vi "Delete FITS.vi"(8 "error in (no error)":errorcluster, 11 "Save Image in":refnum<class "Save Image.lvclass">) -> (0 "error out":errorcluster, 3 "Save Image out":refnum<class "Save Image.lvclass">)   [LabVIEW 2018, in "Save Image.lvclass"]
uses:
  Save Image.lvclass
  Save Image.lvclass/Save Image.ctl
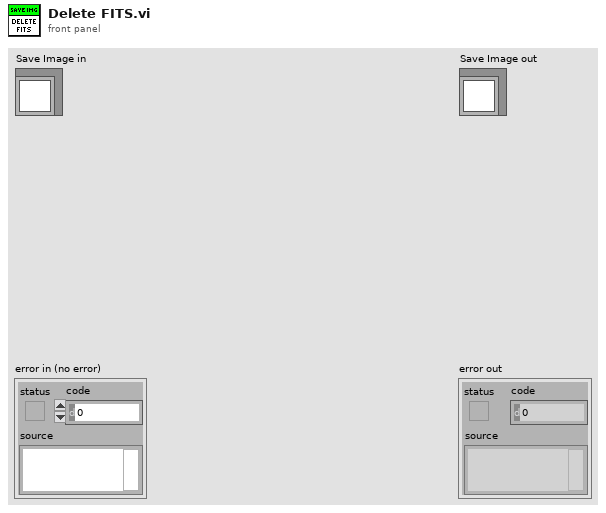
[diagram p1: front panel]
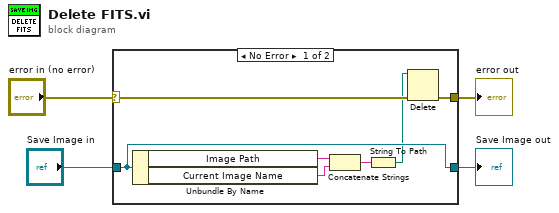
[diagram p0: block diagram]
diagram:
  n1 = case shown="No Error" "error in (no error)" {
    selector: "error in (no error)" -> [w10 w13]
    tunnel: [w9 w13] -> w3
    tunnel: [w11 w12] -> w1
    tunnel: "Save Image in" -> [w11 w12]
    frame No Error {
      n2 = Unbundle By Name(w11) -> ("Image Path"=w7:string, "Current Image Name"=w8:string)
      n3 = Concatenate Strings(w7, w8) -> (w6:string)
      n4 = String To Path(string=w6) -> (path=w5:path)
      n5 = Delete(path (use dialog)=w5, error in=w10) -> (error out=w9:errorcluster)  [unwired: 3 in, 2 out]
    }
    frame Error {
    }
  }
  "error out" <- w3
  "Save Image out" <- w1
